vi "scaleFeaturesPositions_um_pix.vi"(8 "error in (no error)":errorcluster, 9 "dXY":sgl, 10 "dZ":dbl, 11 "FEATURES(µm)":sgl[][](array[numeric])) -> (0 "error out":errorcluster, 3 "Features(pix)":sgl[][](array[numeric]))   [LabVIEW 2023, in "holoTracker.lvlib"]
uses:
  HoloTrackerLib/holoTracker.lvlib
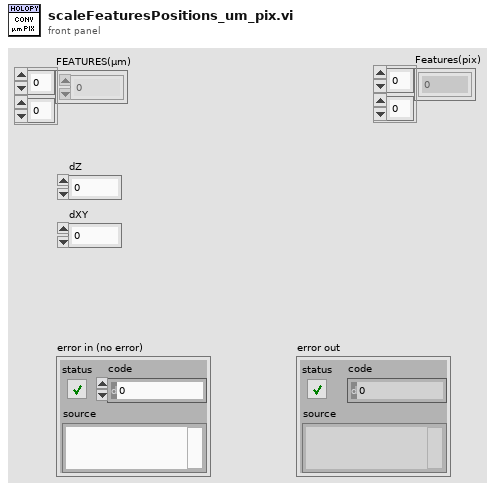
[diagram p1: front panel]
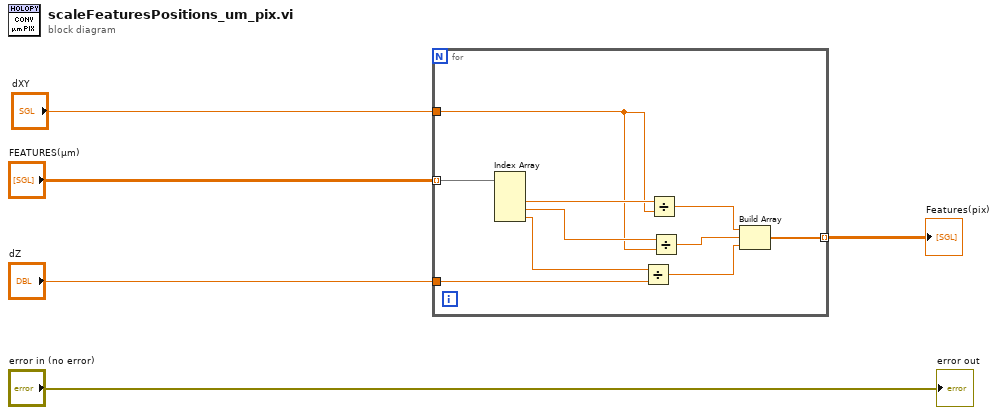
[diagram p0: block diagram]
diagram:
  n1 = for {
    tunnel: "FEATURES(µm)" -> [w15] mode=indexing
    tunnel: [w10] -> w5 mode=indexing
    tunnel: "dXY" -> [w9]
    tunnel: "dZ" -> [w7]
    n2 = Index Array(array=w15) -> (element #2=w14:sgl, element #3=w13:sgl, element #4=w8:sgl)  [unwired: 4 in, 1 out]
    n3 = Divide(x=w8, y=w7) -> (x/y=w6:dbl)
    n4 = Divide(x=w14, y=w9) -> (x/y=w12:sgl)
    n5 = Divide(x=w13, y=w9) -> (x/y=w11:sgl)
    n6 = Build Array(w12, w11, w6) -> (w10:dbl[])
  }
  "Features(pix)" <- w5
  "error out" <- "error in (no error)"
